vi "Open Clearpath Ports.vi"(8 "error in (no error)":errorcluster, 11 "ComPortHub":u64) -> (0 "error out":errorcluster, 2 "ComHubPortOut":refnum<k24>, 3 "m_SzsMgrOut":refnum<k24>)   [LabVIEW 2020]
uses:
  C:/Users/Jonathan/Documents/Clearpath SDK/CSharp Examples/CLRWrapper/x64/Debug/CLRWrapper.dll
  CSharp Examples/CLRWrapper/x64/Debug/CLRWrapper.dll
panel:
  out "NodeCount":u16
  out "OpenState":i32(ring) items=["UNKNOWN", "CLOSED", "FLASHING", "PORT_UNAVAILABLE", "OPENED_SEARCHING", "OPENED_ONLINE"]
  out "NetNumber":u16
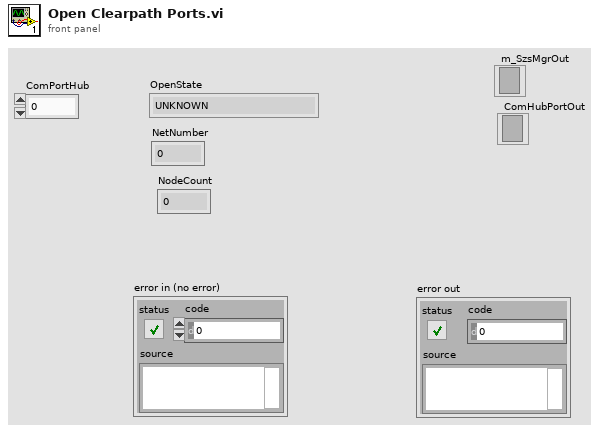
[diagram p1: front panel]
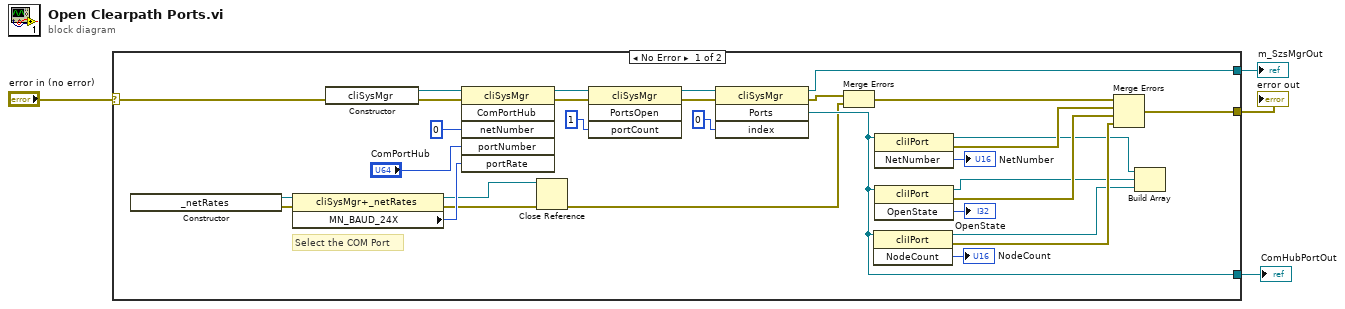
[diagram p0: block diagram]
diagram:
  n1 = case shown="No Error" "error in (no error)" {
    selector: "error in (no error)" -> [w23 w36]
    tunnel: [w9 w36] -> w4
    tunnel: [w22 _] -> w2
    tunnel: [w5 _] -> w1
    frame No Error {
      # "Select the COM Port"
      n2 = constructor class="cliSysMgr+_netRates"() -> (reference out=w33:refnum<k24>, error out=w16:errorcluster)  [unwired: 3 in, 1 out]
      n3 = property class="cliSysMgr+_netRates"(reference=w33, error in=w16) -> (reference out=w18:refnum<k24>, error out=w17:errorcluster, "MN_BAUD_24X"=w32:i32)
      n4 = constructor class="cliSysMgr"(error in=w23) -> (reference out=w29:refnum<k24>, error out=w28:errorcluster)  [unwired: 2 in, 1 out]
      n5 = invoke class="cliSysMgr" method="ComPortHub"(reference=w29, error in=w28, "netNumber"=0, "portNumber"="ComPortHub", "portRate"=w32) -> (reference out=w34:refnum<k24>, error out=w35:errorcluster)  [unwired: 1 in, 4 out]
      n6 = Close Reference(reference=w18, error in (no error)=w17) -> (error out=w11:errorcluster)
      n7 = invoke class="cliSysMgr" method="PortsOpen"(reference=w34, error in=w35, "portCount"=1) -> (reference out=w27:refnum<k24>, error out=w26:errorcluster)  [unwired: 1 in, 2 out]
      n8 = invoke class="cliSysMgr" method="Ports"(reference=w27, error in=w26, "index"=0) -> (reference out=w5:refnum<k24>, error out=w12:errorcluster, "Ports"=w22:refnum<k24>)  [unwired: 1 in, 1 out]
      n9 = Merge Errors(w12, w11) -> (w10:errorcluster)
      n10 = invoke class="cliIPort" method="NodeCount"(reference=w22) -> (reference out=w6:refnum<k24>, error out=w13:errorcluster, "NodeCount"=→"NodeCount":u16)  [unwired: 2 in]
      n11 = invoke class="cliIPort" method="NetNumber"(reference=w22) -> (reference out=w8:refnum<k24>, error out=w15:errorcluster, "NetNumber"=→"NetNumber":u16)  [unwired: 2 in]
      n12 = invoke class="cliIPort" method="OpenState"(reference=w22) -> (reference out=w7:refnum<k24>, error out=w14:errorcluster, "OpenState"=→"OpenState":i32)  [unwired: 2 in]
      n13 = Merge Errors(w10, w15, w14, w13) -> (w9:errorcluster)
      n14 = Build Array(w8, w7, w6) -> ()  [unwired: 1 out]
    }
    frame Error {
    }
  }
  "error out" <- w4
  "ComHubPortOut" <- w2
  "m_SzsMgrOut" <- w1
